vi "测试-按行输入到word报表.vi"() -> ()   [LabVIEW 2018]
uses:
  <vilib>/Utility/NIReport.llb/Report Type.ctl
  <vilib>/Utility/NIReport.llb/Append Report Text (str wrap).vi
  <vilib>/addons/_office/word.llb/Word Edit Cell ([dbl]).vi
  <vilib>/Utility/NIReport.llb/NI_report.lvclass
  <vilib>/Utility/NIReport.llb/Word/NI_Word.lvclass
  <vilib>/addons/_office/NI_ReportGenerationToolkit.lvlib
  <vilib>/Utility/NIReport.llb/NI_ReportGenerationCore.lvlib
  <vilib>/addons/_office/word.llb/Word Edit Cell ([str]).vi
panel:
  out "报表进度":dbl
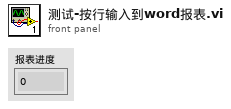
[diagram p1: front panel]
types:
  T1 = cluster{"position (Excel)":cluster{"row":i32, "column":i32}, "name (Excel)":string, "bookmark (Word)":string}
  T2 = typedef "NI_ReportGenerationCore.lvlib/Report Type.ctl" = enum16{"HTML", "Word", "Excel"}
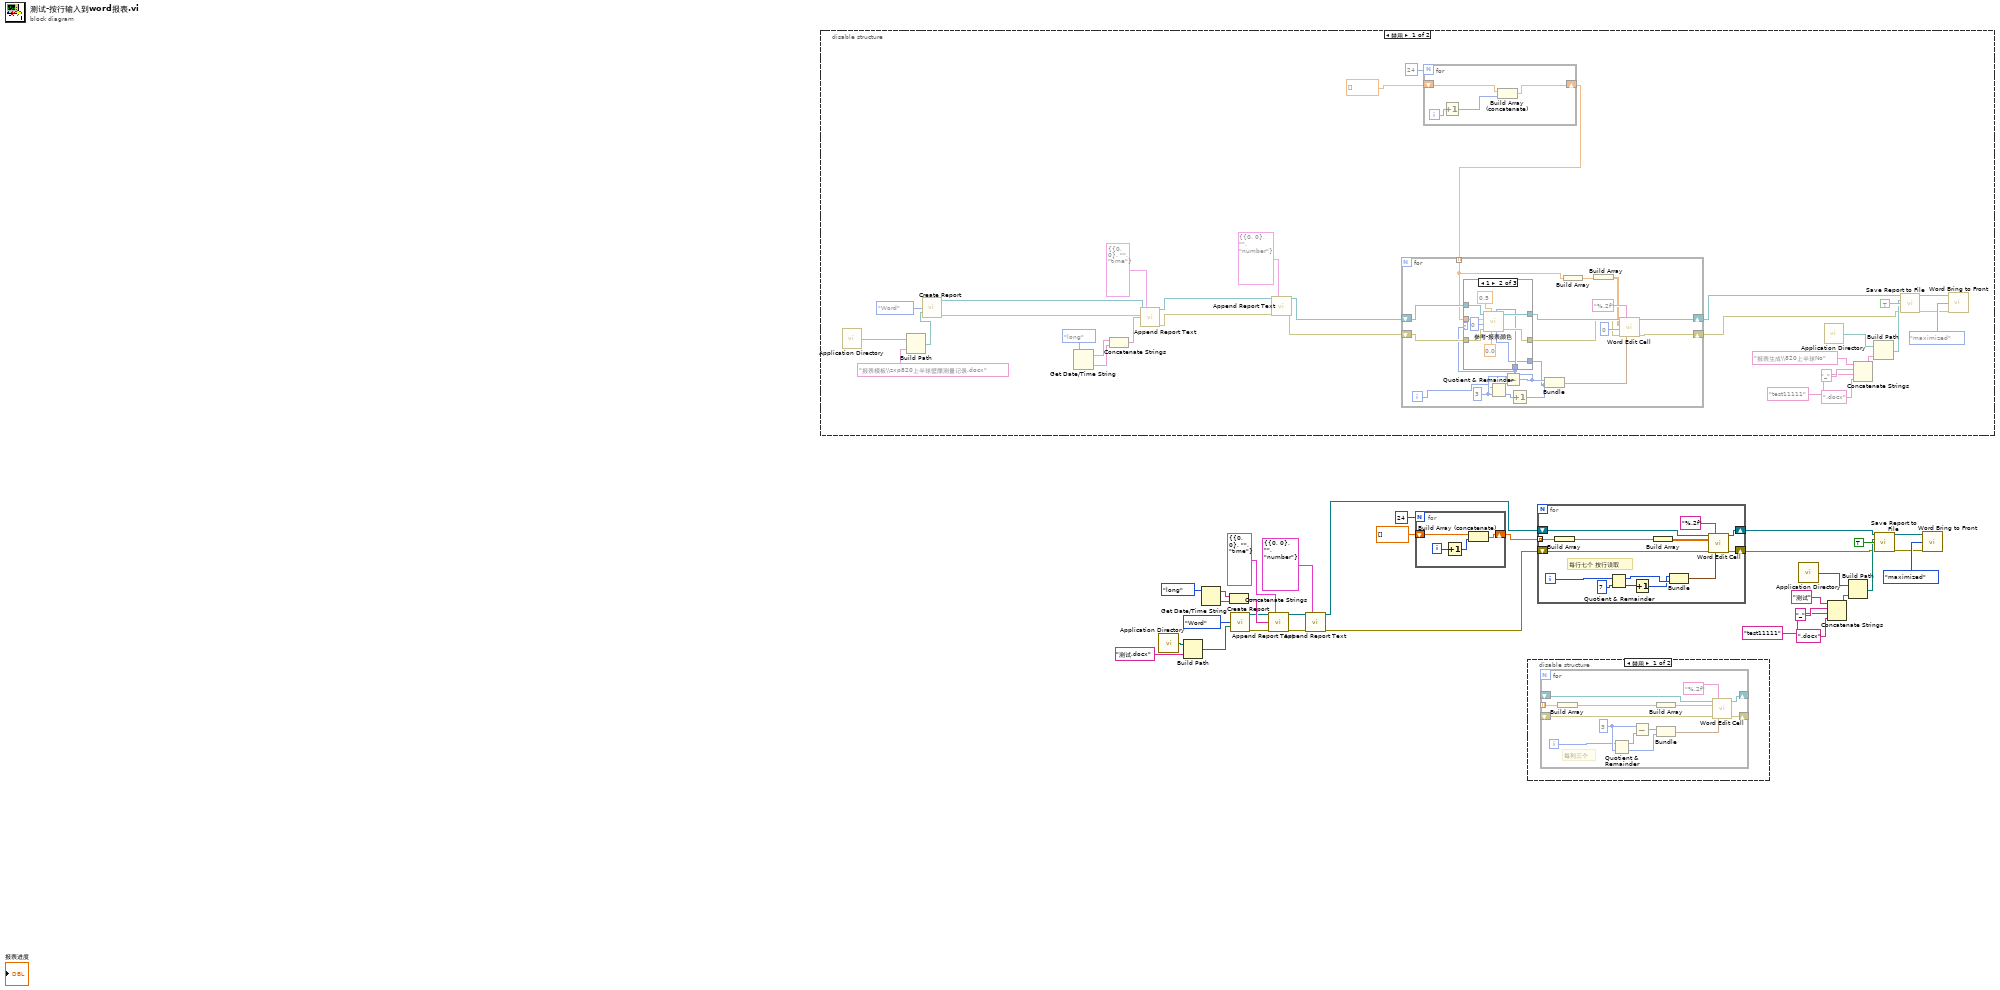
[diagram p0: block diagram]
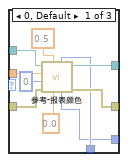
[diagram p3: hidden frame]
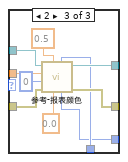
[diagram p4: hidden frame]
diagram:
  n1 = disable-structure shown="禁用" {
    frame Disabled {
      n2 = call <vilib>:"Application Directory.vi"() -> ("Application Directory"=w62:path)
      n3 = Build Path(base path=w62, name or relative path="报表模板\\zxp820上半球壁厚测量记录.docx") -> (appended path=w59:path)
      n4 = call <vilib>:"Create Report.vi"("report type"=Report_Type."Word" ("Report Type"), "template (empty)"=w59) -> ("report out"=w43:refnum<class "NI_report.lvclass">, "error out"=w42:errorcluster)  [unwired: 12 in]
      n5 = Get Date/Time String(date format (0)=enum16{"short", "long", "abbreviated"}."long" ("日期格式(0)")) -> (date string=w58:string, time string=w56:string)  [unwired: 2 in]
      n6 = Concatenate Strings(w58, w56) -> (w57:string)
      n7 = call-poly <vilib>:"Append Report Text.vi"("report in"=w43, "MS Office parameters"=T1 {"position (Excel)"={"row"=0, "column"=0}, "name (Excel)"="", "bookmark (Word)"="time"}, "text"=w57, "error in (no error)"=w42) -> ("report out"=w40:refnum<class "NI_report.lvclass">, "error out"=w39:errorcluster)  [unwired: 8 in, 2 out]
      n8 = call-poly <vilib>:"Append Report Text.vi"("report in"=w40, "MS Office parameters"=T1 {"position (Excel)"={"row"=0, "column"=0}, "name (Excel)"="", "bookmark (Word)"="number"}, "error in (no error)"=w39) -> ("report out"=w38:refnum<class "NI_report.lvclass">, "error out"=w37:errorcluster)  [unwired: 9 in, 2 out]
      n9 = for {
        N: 24 -> [_]
        shift-right: [w115] -> w34
        shift-left: dbl[] [] -> [w116]
        i -> [w114]
        n10 = Increment(x=w114) -> (x+1=w113:i32)
        n11 = Build Array (concatenate)(w116, w113) -> (w115:dbl[])
      }
      n12 = for {
        shift-right: [w81] -> w36
        shift-left: w38 -> [w78]
        shift-right: [w80] -> w35
        shift-left: w37 -> [w77]
        tunnel: w34 -> [w74] mode=indexing
        i -> [w65]
        w69 = 3 ("y")
        n13 = Quotient & Remainder(x=w65, y=w69) -> (x-y*floor(x/y)=w70:i32, floor(x/y)=w67:i32)
        n14 = Subtract(x=w69, y=w70) -> (x-y=w68:i32)
        n15 = Increment(x=w67) -> (x+1=w66:i32)
        n16 = case shown="1" w68 {
          tunnel: w78 -> [w92 w102 w112]
          tunnel: [w91 w101 w111] -> w76
          tunnel: [w90 w100 w110] -> w75
          tunnel: w77 -> [w89 w99 w109]
          tunnel: w74 -> [w86 w96 w106]
          tunnel: w68 -> [w85 w95 w105]
          tunnel: w66 -> [w84 w94 w104]
          frame 0, Default {
            n17 = call "参考-报表颜色.vi"("列"=w84, "行"=w85, "下限"=0.0, "上限"=0.5, "error in (no error)"=w89, "table index (-1)"=i16 0, "厚度值"=w86, "report in"=w92) -> ("error out"=w90:errorcluster, "report out"=w91:refnum<class "NI_report.lvclass">)  [unwired: 2 in]
          }
          frame 1 {
            n18 = call "参考-报表颜色.vi"("列"=w94, "行"=w95, "下限"=0.0, "上限"=0.5, "error in (no error)"=w99, "table index (-1)"=i16 0, "厚度值"=w96, "report in"=w102) -> ("error out"=w100:errorcluster, "report out"=w101:refnum<class "NI_report.lvclass">)  [unwired: 2 in]
          }
          frame 2 {
            n19 = call "参考-报表颜色.vi"("列"=w104, "行"=w105, "下限"=0.0, "上限"=0.5, "error in (no error)"=w109, "table index (-1)"=i16 0, "厚度值"=w106, "report in"=w112) -> ("error out"=w110:errorcluster, "report out"=w111:refnum<class "NI_report.lvclass">)  [unwired: 2 in]
          }
        }
        n20 = Bundle(w68, w66) -> (w71:cluster{i32, i32})  [unwired: 1 in]
        n21 = Build Array(w74) -> (w73:dbl[])
        n22 = Build Array(w73) -> (w72:dbl[][])
        n23 = call-poly <vilib>:"Word Edit Cell.vi"("report in"=w76, "format string (%.3f)"="%.2f", "value"=w72, "table index (-1)"=i16 0, "error in (no error)"=w75, "start (0, 0)"=w71) -> ("report out"=w81:refnum<class "NI_report.lvclass">, "error out"=w80:errorcluster)  [unwired: 8 in]
      }
      n24 = call <vilib>:"Application Directory.vi"() -> ("Application Directory"=w51:path)
      n25 = Concatenate Strings("报表生成\\820上半球No" ("字符串"), "_" ("名称或相对路径"), "test11111" ("字符串"), ".docx" ("名称或相对路径")) -> (w50:string)
      n26 = Build Path(base path=w51, name or relative path=w50) -> (appended path=w52:path)
      n27 = call-dynamic "Save Report to File.vi"("report in"=w36, "report file path"=w52, "prompt to replace? (F)"=TRUE, "error in (no error)"=w35) -> ("report out"=w45:refnum<class "NI_report.lvclass">, "error out"=w44:errorcluster)  [unwired: 10 in]
      n28 = call <vilib>:"Word Bring to Front.vi"("report in"=w45, "window state (maximized)"=enum16{"maximized", "minimized", "normal"}."maximized", "error in (no error)"=w44) -> ()  [unwired: 11 in, 2 out]
    }
    frame Enabled {
    }
  }
  n29 = call <vilib>:"Application Directory.vi"() -> ("Application Directory"=w30:path)
  n30 = Build Path(base path=w30, name or relative path="测试.docx") -> (appended path=w27:path)
  n31 = Get Date/Time String(date format (0)=enum16{"short", "long", "abbreviated"}."long" ("日期格式(0)")) -> (date string=w26:string, time string=w24:string)  [unwired: 2 in]
  n32 = Concatenate Strings(w26, w24) -> (w25:string)
  n33 = call <vilib>:"Create Report.vi"("report type"=Report_Type."Word" ("Report Type"), "template (empty)"=w27) -> ("report out"=w11:refnum<class "NI_report.lvclass">, "error out"=w10:errorcluster)  [unwired: 12 in]
  n34 = call-poly <vilib>:"Append Report Text.vi"("report in"=w11, "MS Office parameters"=T1 {"position (Excel)"={"row"=0, "column"=0}, "name (Excel)"="", "bookmark (Word)"="time"}, "text"=w25, "error in (no error)"=w10) -> ("report out"=w8:refnum<class "NI_report.lvclass">, "error out"=w7:errorcluster)  [unwired: 8 in, 2 out]
  n35 = call-poly <vilib>:"Append Report Text.vi"("report in"=w8, "MS Office parameters"=T1 {"position (Excel)"={"row"=0, "column"=0}, "name (Excel)"="", "bookmark (Word)"="number"}, "error in (no error)"=w7) -> ("report out"=w6:refnum<class "NI_report.lvclass">, "error out"=w5:errorcluster)  [unwired: 9 in, 2 out]
  n36 = for {
    N: 24 -> [_]
    shift-right: [w119] -> w2
    shift-left: dbl[] [] -> [w120]
    i -> [w118]
    n37 = Increment(x=w118) -> (x+1=w117:i32)
    n38 = Build Array (concatenate)(w120, w117) -> (w119:dbl[])
  }
  n39 = disable-structure shown="禁用" {
    frame Disabled {
      n40 = for {
        shift-right: [w134] -> _
        shift-left: _ -> [w123]
        shift-right: [w133] -> _
        shift-left: _ -> [w122]
        tunnel: _ -> [w131] mode=indexing
        i -> [w124]
        w126 = 3 ("y")
        # "每列三个"
        n41 = Build Array(w131) -> (w130:void[])
        n42 = Quotient & Remainder(x=w124, y=w126) -> (x-y*floor(x/y)=w127:i32, floor(x/y)=w121:i32)
        n43 = Subtract(x=w126, y=w127) -> (x-y=w125:i32)
        n44 = Build Array(w130) -> (w129:void[])
        n45 = Bundle(w125, w121) -> (w128:cluster{i32, i32})  [unwired: 1 in]
        n46 = call-poly <vilib>:"Word Edit Cell.vi"("report in"=w123, 1:"%.2f" ("format string (%.3f)"), "value"=w129, "error in (no error)"=w122, "start (0, 0)"=w128) -> ("report out"=w134:refnum<class "NI_report.lvclass">, "error out"=w133:errorcluster)  [unwired: 9 in]
      }
    }
    frame Enabled {
    }
  }
  n47 = for {
    shift-right: [w148] -> w4
    shift-left: w6 -> [w139]
    shift-right: [w147] -> w3
    shift-left: w5 -> [w138]
    tunnel: w2 -> [w145] mode=indexing
    i -> [w140]
    # "每行七个 按行读取"
    n48 = Build Array(w145) -> (w144:dbl[])
    n49 = Quotient & Remainder(x=w140, y=7) -> (x-y*floor(x/y)=w137:i32, floor(x/y)=w136:i32)
    n50 = Increment(x=w136) -> (x+1=w135:i32)
    n51 = Build Array(w144) -> (w143:dbl[][])
    n52 = Bundle(w135, w137) -> (w142:cluster{i32, i32})  [unwired: 1 in]
    n53 = call-poly <vilib>:"Word Edit Cell.vi"("report in"=w139, "format string (%.3f)"="%.2f", "value"=w143, "error in (no error)"=w138, "start (0, 0)"=w142) -> ("report out"=w148:refnum<class "NI_report.lvclass">, "error out"=w147:errorcluster)  [unwired: 9 in]
  }
  n54 = call <vilib>:"Application Directory.vi"() -> ("Application Directory"=w19:path)
  n55 = Concatenate Strings("测试" ("字符串"), "_" ("名称或相对路径"), "test11111" ("字符串"), ".docx" ("名称或相对路径")) -> (w18:string)
  n56 = Build Path(base path=w19, name or relative path=w18) -> (appended path=w20:path)
  n57 = call-dynamic "Save Report to File.vi"("report in"=w4, "report file path"=w20, "prompt to replace? (F)"=TRUE, "error in (no error)"=w3) -> ("report out"=w13:refnum<class "NI_report.lvclass">, "error out"=w12:errorcluster)  [unwired: 10 in]
  n58 = call <vilib>:"Word Bring to Front.vi"("report in"=w13, "window state (maximized)"=enum16{"maximized", "minimized", "normal"}."maximized", "error in (no error)"=w12) -> ()  [unwired: 11 in, 2 out]
